vi "DCMotorSim_example.vi"() -> ()   [LabVIEW 2019]
uses:
  <vilib>/Rock Robotics/WPI/ThirdParty/JAS_Junk/TrajLib/Enum/DCMOTOR_TYPES_ENUM.ctl
  <vilib>/Rock Robotics/WPI/ThirdParty/JAS_Junk/TrajLib/BatterySim_CalculateLoadedBatteryVoltage.vi
  <vilib>/Rock Robotics/WPI/ThirdParty/JAS_Junk/TrajLib/Trajectory_Library.lvlib
  <vilib>/Analysis/Matrix/Datatypes/RealMatrix.ctl
  <vilib>/Analysis/Matrix/NI_Matrix.lvlib
  <vilib>/Rock Robotics/WPI/ThirdParty/JAS_Junk/TrajLib/TypeDef/LINEAR_SYSTEM.ctl
  <vilib>/Rock Robotics/WPI/ThirdParty/JAS_Junk/TrajLib/TypeDef/LINEAR_SYSTEM_SIM.ctl
  <vilib>/Rock Robotics/WPI/ThirdParty/JAS_Junk/TrajLib/TypeDef/DCMOTOR.CTL
  <vilib>/Rock Robotics/WPI/ThirdParty/JAS_Junk/TrajLib/TypeDef/DCMOTOR_SIM.ctl
panel:
  in  "Tab Control":enum32{"Control", "Simulation"}(tab)
  in  "Motor Dmd - SP\n( +/- 1 )":dbl(slide) scale=-1.0..1.0
  out "Motor Speed - PV (RPM)":dbl format="%20.3f"
  out "Battery Voltage (Volts)":dbl format="%20.3f"
  out "Voltage, Current Chart":cluster{dbl, "Voltage":dbl}(graph)
  out "PV, SP Chart":T1(graph)
  out "Motor Current (Amps)":dbl format="%20.3f"
  out "Motor Position (Rotations)":dbl format="%20.3f"
  out "DcMotorSim":T2 {"GearBox"."Jr_KgM2" format="%13.5p"; "GearBox"."L_H" format="%13.5p"; "GearBox"."Kt_NMPerAmp" format="%13.5p"; "GearBox"."KvINV_RadPerSecPerVolt" format="%13.5p"; "GearBox"."R_Ohms" format="%13.5p"; "GearBox"."FreeSpeed_RadPerSec" format="%13.5p"; "GearBox"."FreeCurrent_Amps" format="%13.5p"; "GearBox"."StallCurrent_Amps" format="%13.5p"; "GearBox"."StallTorque_NM" format="%13.5p"; "GearBox"."nominalVoltage_Volts" format="%13.5p"}
  # "<States, 1>"
  # "<Outputs, 1>"
  # "<Inputs, 1>"
  # "<Outputs, 1>"
  # "<States,States>"
  # "<States,Inputs>"
  # "<Outputs,States>"
  # "<Outputs,Inputs>"
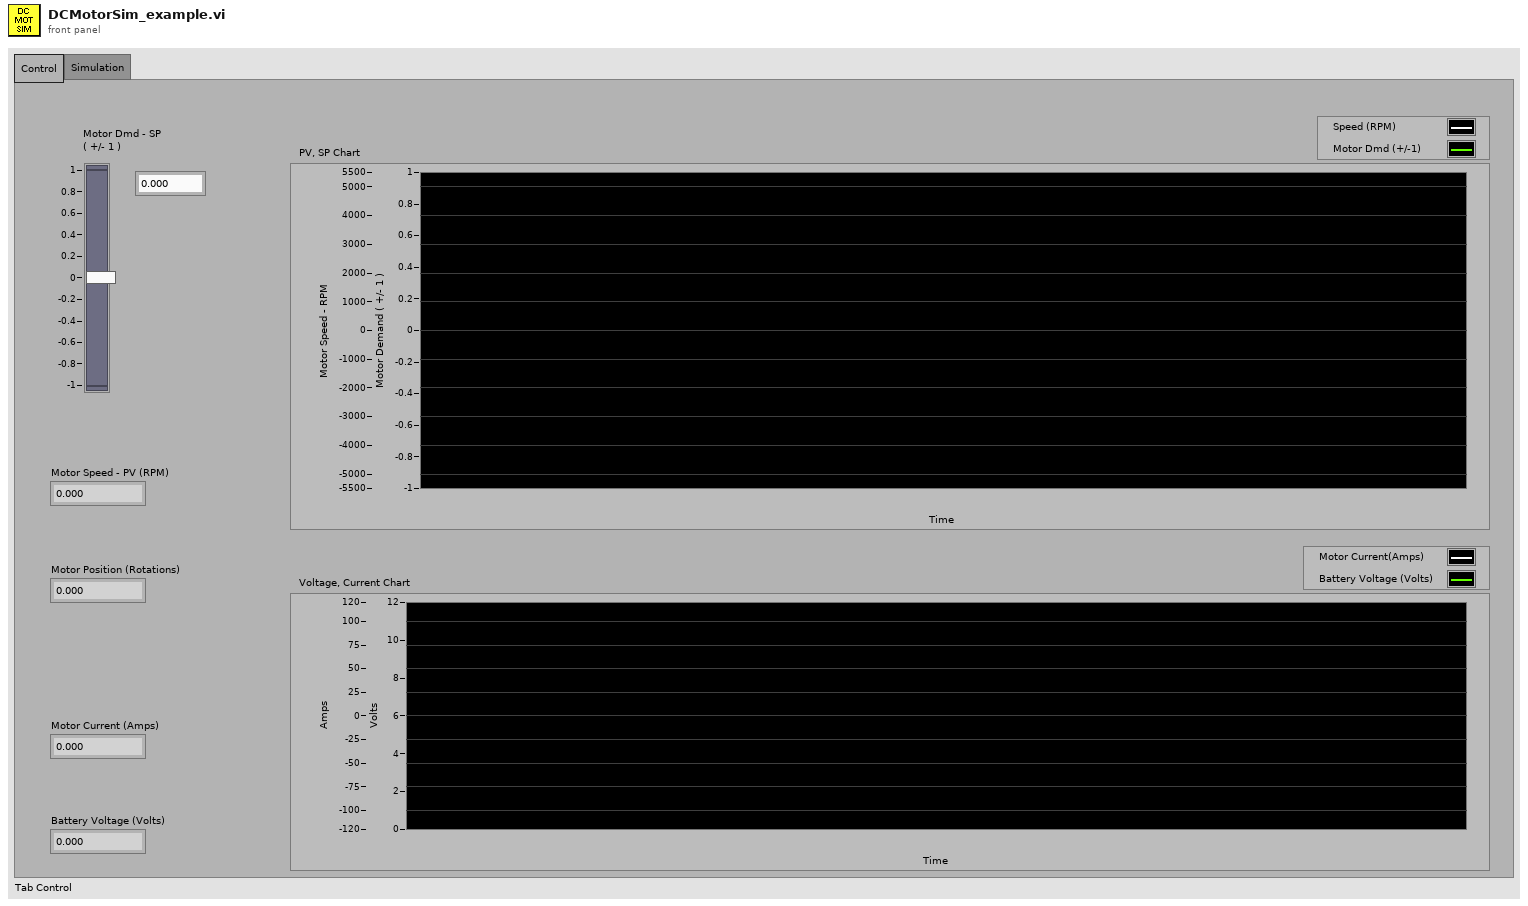
[diagram p1: front panel]
types:
  T1 = cluster{"Velocity_RPM":dbl, "Motor Dmd - SP\n( +/- 1 )":dbl}
  T2 = typedef "Trajectory_Library.lvlib/DCMOTOR_SIM.ctl" = cluster{"LinearSystemSim":T3, "GearBox":T6, "Gearing":dbl}
  T3 = typedef "Trajectory_Library.lvlib/LINEAR_SYSTEM_SIM.ctl" = cluster{"m_Plant":T4, "m_X":T5, "m_Y":T5, "m_U":T5, "MeasureStdDev":T5}
  T4 = typedef "Trajectory_Library.lvlib/LINEAR_SYSTEM.ctl" = cluster{"m_A":T5, "m_B":T5, "m_C":T5, "m_D":T5, "States":i32, "Inputs":i32, "Outputs":i32}
  T5 = typedef "NI_Matrix.lvlib/RealMatrix.ctl" = dbl[][]
  T6 = typedef "Trajectory_Library.lvlib/DCMOTOR.CTL" = cluster{"nominalVoltage_Volts":dbl, "StallTorque_NM":dbl, "StallCurrent_Amps":dbl, "FreeCurrent_Amps":dbl, "FreeSpeed_RadPerSec":dbl, "R_Ohms":dbl, "KvINV_RadPerSecPerVolt":dbl, "Kt_NMPerAmp":dbl, "L_H":dbl, "Jr_KgM2":dbl}
  T7 = typedef "Trajectory_Library.lvlib/DCMOTOR_TYPES_ENUM.ctl" = enum16{"CIM", "AndyMark 9015", "Andy Mark RS 775 125", "Bag", "BaneBots RS 550", "BaneBots RS 775", "Falcon 500", "Mini CIM", "NEO", "NEO 550", "Romi BuiltIn", "Vex 775 Pro", "Snow Blower AM 2235A", "Bosch Seat AM 3493"}
  T8 = typedef "Trajectory_Library.lvlib/LINEAR_SYSTEM_ID_DCMOTOR_MODEL.ctl" = cluster{"DCMOTOR_TYPES":T7, "Num Motors":i32, "Gearing":dbl, "MOI kgm2":dbl}
  T9 = typedef "Trajectory_Library.lvlib/DCMOTOR_SIM_SIMULATION_PARAMS.ctl" = cluster{"Pos Sim Std Dev Rotations":dbl, "Vel Sim Std Dev RPM":dbl}
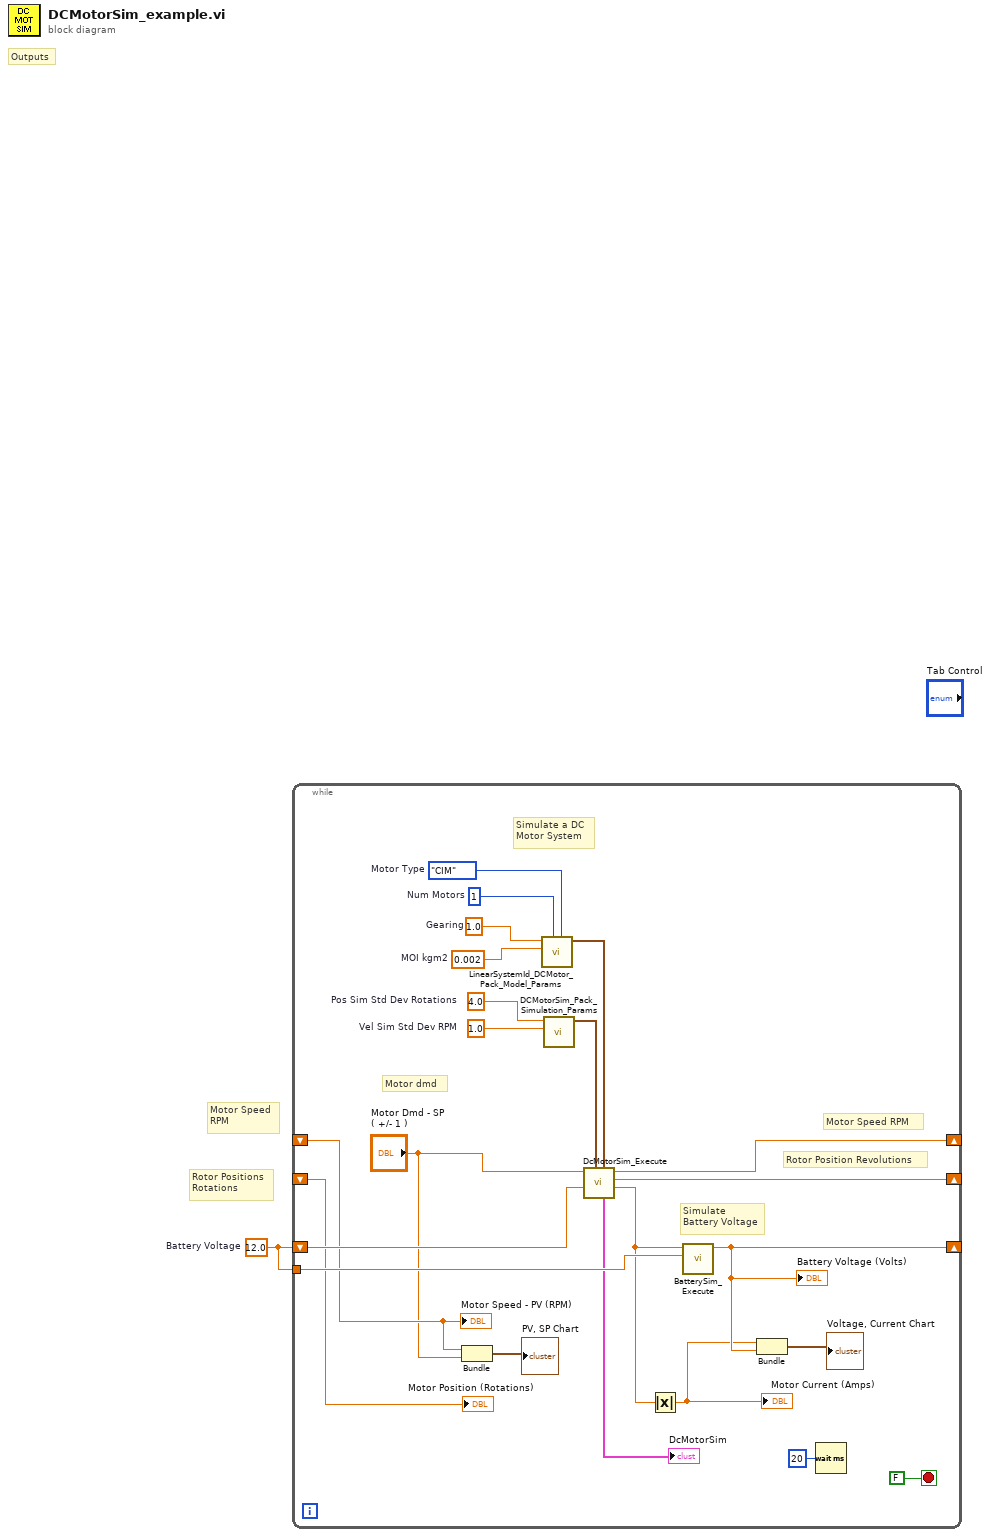
[diagram p0: block diagram]
diagram:
  w1 = 12.0  # Battery Voltage
  # "Rotor Positions\nRotations"
  # "Motor Speed\nRPM"
  # "Outputs"
  n1 = while {
    shift-right: [w4] -> _
    shift-left: w1 -> [w17]
    shift-right: [w18] -> _
    shift-left: _ -> [w9]
    shift-right: [w15] -> _
    shift-left: _ -> [w8]
    tunnel: w1 -> [w11]
    stop <- FALSE stop-if-true
    w12 = 4.0  # Pos Sim Std Dev Rotations
    w13 = 1.0  # Vel Sim Std Dev RPM
    w21 = 1.0  # Gearing
    w22 = 0.002  # MOI kgm2
    w23 = 1  # Num Motors
    w24 = DCMOTOR_TYPES_ENUM."CIM"  # Motor Type
    # "Motor dmd"
    # "Rotor Position Revolutions"
    # "Motor Speed RPM"
    # "Simulate\nBattery Voltage"
    # "Simulate a DC \nMotor System"
    n2 = Bundle("Velocity_RPM"=w9, "Motor Dmd - SP\n( +/- 1 )"="Motor Dmd - SP\n( +/- 1 )") -> (→"PV, SP Chart":T1)  [unwired: 1 in]
    n3 = call <vilib>:"LinearSystemId_DCMotor_Pack_Model_Params.vi"("DCMOTOR_TYPES"=w24, "Num Motors"=w23, "MOI kgm2"=w22, "Gearing"=w21) -> ("LinearSystem_ID_DCMotor_Model"=w16:T8)  [unwired: 7 in]
    n4 = call <vilib>:"DCMotorSim_Pack_Simulation_Params.vi"("Vel Sim Std Dev RPM"=w13, "Pos Sim Std Dev Rotations"=w12) -> ("DCMOTOR_Sim_Simulation_Params"=w14:T9)  [unwired: 9 in]
    n5 = call <vilib>:"DcMotorSim_Execute.vi"("DCMotor_Model _Params"=w16, "DCMOTORSim_Simulation_Params"=w14, "Battery Voltage"=w17, "Motor Dmd (CO)"="Motor Dmd - SP\n( +/- 1 )") -> ("Motor Current"=w6:dbl, "Position_Rotations"=w15:dbl, "Velocity_RPM"=w18:dbl, "out DcMotorSim"=→"DcMotorSim":T2)  [unwired: 3 in, 1 out]
    n6 = Absolute Value(x=w6) -> (abs(x)=w3:dbl)
    "Motor Current (Amps)" <- w3
    n7 = call <vilib>:"BatterySim_Execute.vi"("Nominal Battery Voltage"=w11, "Current"=w6) -> ("Voltage"=w4:dbl)  [unwired: 9 in]
    "Battery Voltage (Volts)" <- w4
    n8 = Bundle(w3, "Voltage"=w4) -> (→"Voltage, Current Chart":cluster{dbl, "Voltage":dbl})  [unwired: 1 in]
    n9 = Wait (ms)(milliseconds to wait=u32 20) -> ()  [unwired: 1 out]
    "Motor Speed - PV (RPM)" <- w9
    "Motor Position (Rotations)" <- w8
  }
